vi "FlatToRichni_xnet_can_bm_api_InitializeSettingsRequest.vi"(5 "OutputClusterType":T1, 11 "InputCluster":T6) -> (3 "OutputCluster":T1)   [LabVIEW 2025, in "xnet_can_bus_monitor_api_client.lvlib"]
uses:
  ni_xnet_can_bm_api_InitializeSettingsRequest_Flat.ctl
  ni_xnet_can_bm_api_ConnectSettings_Flat.ctl
  ni_xnet_can_bm_api_CanMode.ctl
  ni_xnet_can_bm_api_Termination.ctl
  ni_xnet_can_bm_api_FdIsoMode.ctl
  ni_xnet_can_bm_api_InitializeSettingsRequest.ctl
  ni_xnet_can_bm_api_ConnectSettings.ctl
  xnet_can_bus_monitor_api_client.lvlib
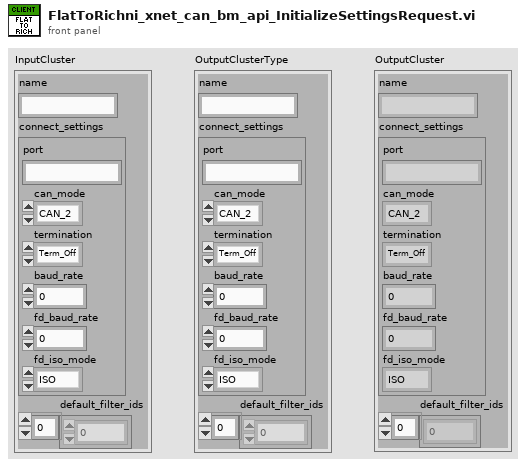
[diagram p1: front panel]
types:
  T1 = typedef "xnet_can_bus_monitor_api_client.lvlib/ni_xnet_can_bm_api_InitializeSettingsRequest.ctl" = cluster{"name":string, "connect_settings":T2, "default_filter_ids":u32[]}
  T2 = typedef "xnet_can_bus_monitor_api_client.lvlib/ni_xnet_can_bm_api_ConnectSettings.ctl" = cluster{"port":string, "can_mode":T3, "termination":T4, "baud_rate":u64, "fd_baud_rate":u64, "fd_iso_mode":T5}
  T3 = typedef "xnet_can_bus_monitor_api_client.lvlib/ni_xnet_can_bm_api_CanMode.ctl" = enum32{"CAN_2", "CAN_FD", "CAN_FD_BRS"}
  T4 = typedef "xnet_can_bus_monitor_api_client.lvlib/ni_xnet_can_bm_api_Termination.ctl" = enum32{"Term_Off", "Term_On"}
  T5 = typedef "xnet_can_bus_monitor_api_client.lvlib/ni_xnet_can_bm_api_FdIsoMode.ctl" = enum32{"ISO", "Non_ISO", "ISO_Legacy"}
  T6 = typedef "xnet_can_bus_monitor_api_client.lvlib/ni_xnet_can_bm_api_InitializeSettingsRequest_Flat.ctl" = cluster{"name":string, "connect_settings":T7, "default_filter_ids":u32[]}
  T7 = typedef "xnet_can_bus_monitor_api_client.lvlib/ni_xnet_can_bm_api_ConnectSettings_Flat.ctl" = cluster{"port":string, "can_mode":T3, "termination":T4, "baud_rate":u64, "fd_baud_rate":u64, "fd_iso_mode":T5}
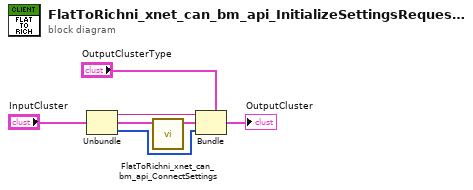
[diagram p0: block diagram]
diagram:
  n1 = Unbundle "Unbundle"("InputCluster") -> ("name"=w4:string, "connect_settings"=w3:T7, "default_filter_ids"=w1:u32[])
  n2 = call "FlatToRichni_xnet_can_bm_api_ConnectSettings.vi"("InputCluster"=w3) -> ("OutputCluster"=w2:T2)  [unwired: 10 in]
  n3 = Bundle "Bundle"(cluster="OutputClusterType", "name"=w4, "connect_settings"=w2, "default_filter_ids"=w1) -> (→"OutputCluster":T1)
